vi "Address Claim Address.vi"(8 "error in":errorcluster, 9 "Names":T1[](array[typedef]), 10 "Requested Addresses":u8[](array[numeric]), 11 "session in":refnum<k21>) -> (0 "error out":errorcluster, 3 "session out":refnum<k21>)   [LabVIEW 2015, in "J1939 Addon Engine.lvlib"]
uses:
  J1939 Addon Engine.lvlib
  Shared/J1939 Utilities/Types/Convert CAN Data (U8) Cluster.ctl
  Shared/J1939 Utilities/Types/CAN Outgoing Message Cluster.ctl
  Shared/J1939 Utilities/Types/PGN Fields Cluster.ctl
  Shared/J1939 Utilities/SubVIs/Convert J1939 ID to CAN Arb ID.vi
  <vilib>/xnet/xnet.llb/XNET Write (Frame CAN).vi
  Shared/J1939 Utilities/J1939 Utilities.lvlib
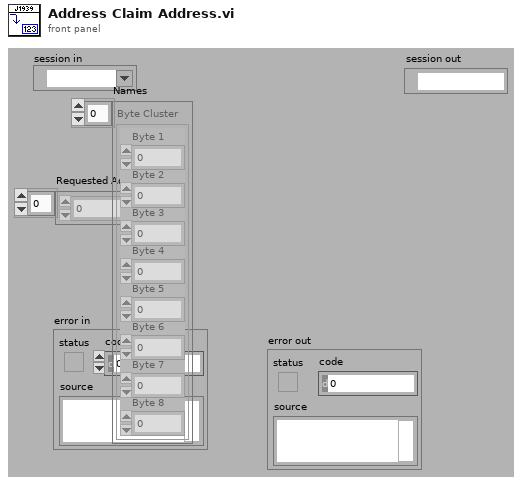
[diagram p1: front panel]
types:
  T1 = typedef "J1939 Addon Shared.lvlib/J1939 Utilities.lvlib/Convert CAN Data (U8) Cluster.ctl" = cluster{"Byte 1":u8, "Byte 2":u8, "Byte 3":u8, "Byte 4":u8, "Byte 5":u8, "Byte 6":u8, "Byte 7":u8, "Byte 8":u8}
  T2 = typedef "J1939 Addon Shared.lvlib/J1939 Utilities.lvlib/PGN Fields Cluster.ctl" = cluster{"Reserved Bit":u8, "Data page":u8, "PDU Format":u8, "PDU Specific":u8}
  T3 = typedef "J1939 Addon Shared.lvlib/J1939 Utilities.lvlib/CAN Outgoing Message Cluster.ctl" = cluster{"Identifier":u32, "Data":u8[]}
  T4 = typedef "XNET Frame CAN.ctl" = cluster{"timestamp":timestamp, "payload":u8[], "identifier":u32, "type":T5, "extended?":bool, "echo?":bool}
  T5 = typedef "XNET Frame Type CAN.ctl" = u8
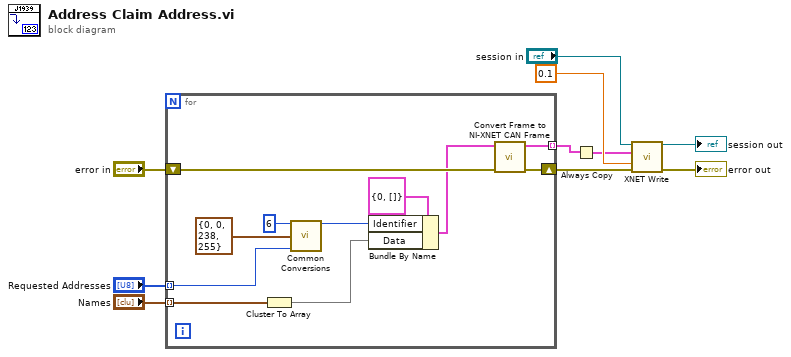
[diagram p0: block diagram]
diagram:
  n1 = for {
    tunnel: "Requested Addresses" -> [w19] mode=indexing
    tunnel: "Names" -> [w11] mode=indexing
    tunnel: [w17] -> w2 mode=indexing
    shift-right: [w13] -> w5
    shift-left: "error in" -> [w16]
    n2 = Cluster To Array(cluster=w11) -> (array=w12:u8[])
    n3 = call-poly "Common Conversions.vi"("Priority"=u8 6, "PGN Fields"=T2 {"Reserved Bit"=0, "Data page"=0, "PDU Format"=238, "PDU Specific"=255}, "Source Address"=w19) -> ("ID"=w20:u32)  [unwired: 2 in, 10 out]
    n4 = Bundle By Name(cluster=T3 {"Identifier"=0, "Data"=[]} ("Data to Send"), "Identifier"=w20, "Data"=w12) -> (w15:T3)
    n5 = call "Convert Frame to NI-XNET CAN Frame.vi"("error in (no error)"=w16, "Data to Send"=w15) -> ("error out"=w13:errorcluster, "CAN frame"=w17:T4)  [unwired: 8 in]
  }
  n6 = Always Copy(1:w2) -> (0:w1:T4[])
  n7 = call-poly <vilib>:"XNET Write.vi"("session in"="session in", "data"=w1, "timeout (10)"=0.1, "error in (no error)"=w5) -> ("session out"=→"session out":refnum<k21>, "error out"=→"error out":errorcluster)  [unwired: 10 out]
